vi "Get Menu Item VI.vi"(7 "Menu Item":string, 8 "error in (no error)":errorcluster, 9 "GUID":string, 10 "Item Ref":T1 format="%.0x", 11 "System Explorer Dispatcher Implementation in":refnum<class "System Explorer Dispatcher.lvclass">) -> (0 "error out":errorcluster, 2 "menu item reference":refnum<vi>, 3 "System Explorer Dispatcher Implementation out":refnum<class "System Explorer Dispatcher.lvclass">)   [LabVIEW 2020, in "Ballard MIL-STD-1553 System Explorer.lvlib" / "Implementation.lvlib" / "System Explorer Dispatcher.lvclass"]
uses:
  System Explorer Dispatcher.lvclass
  Scripting/Constants.vi
  Scripting/Ballard MIL-STD-1553 Scripting.lvlib
  Implementation.lvlib
  <vilib>/NI VeriStand/Custom Device API/Custom Device Item Ref.ctl
  <vilib>/NI VeriStand/Custom Device API/Custom Device API.lvlib
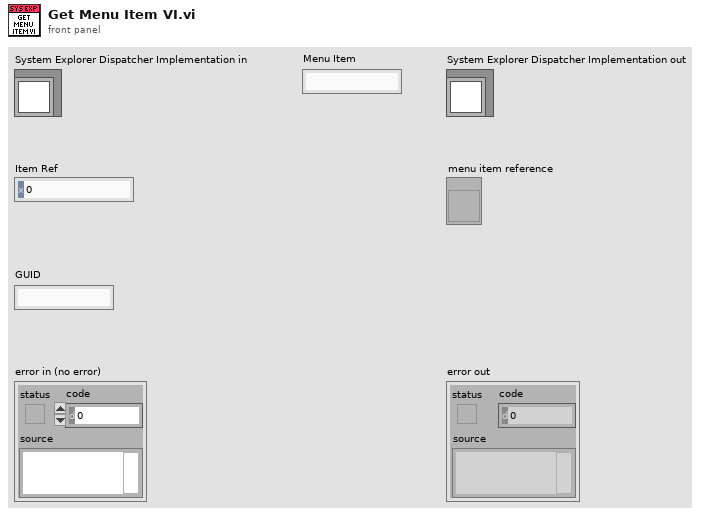
[diagram p1: front panel]
types:
  T1 = typedef "Custom Device API.lvlib/Custom Device Item Ref.ctl" = u64
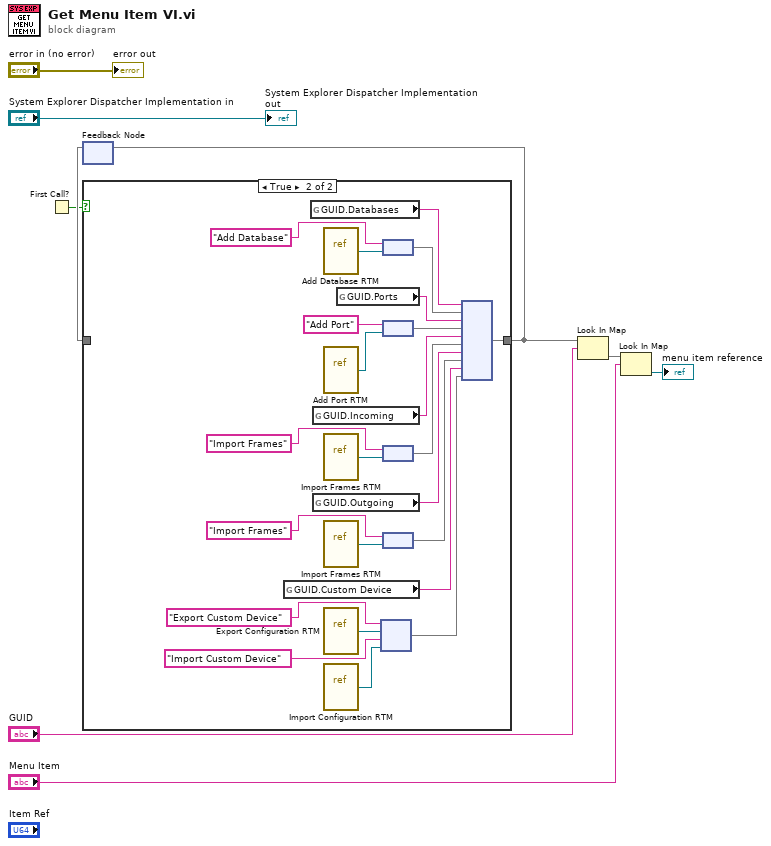
[diagram p0: block diagram]
diagram:
  n1 = First Call?() -> (First Call?: T/F=w1:bool)
  n2 = feedback #1() -> (w7:map{string, map{string, refnum<vi>}})  [unwired: 1 in]
  n3 = case shown="True" w1 {
    tunnel: [w10 w33] -> w8
    tunnel: w7 -> [w10 _]
    frame False {
    }
    frame True {
      n4 = global read "Constants.vi" "GUID.Custom Device"() -> (w14:string)
      n5 = global read "Constants.vi" "GUID.Databases"() -> (w32:string)
      n6 = global read "Constants.vi" "GUID.Incoming"() -> (w22:string)
      n7 = global read "Constants.vi" "GUID.Outgoing"() -> (w18:string)
      n8 = vi-ref "Add Database RTM.vi"() -> (w28:refnum<vi>)
      n9 = vi-ref "Add Port RTM.vi"() -> (w25:refnum<vi>)
      n10 = vi-ref "Import Frames RTM.vi"() -> (w24:refnum<vi>)
      n11 = vi-ref "Import Frames RTM.vi"() -> (w19:refnum<vi>)
      n12 = vi-ref "Export Configuration RTM.vi"() -> (w16:refnum<vi>)
      n13 = vi-ref "Import Configuration RTM.vi"() -> (w11:refnum<vi>)
      n14 = global read "Constants.vi" "GUID.Ports"() -> (w31:string)
      n15 = node("Export Custom Device", w16, "Import Custom Device", w11) -> (w13:map{string, refnum<vi>})
      n16 = node("Add Database", w28) -> (w30:map{string, refnum<vi>})
      n17 = node("Add Port", w25) -> (w26:map{string, refnum<vi>})
      n18 = node("Import Frames", w24) -> (w21:map{string, refnum<vi>})
      n19 = node("Import Frames", w19) -> (w17:map{string, refnum<vi>})
      n20 = node(w32, w30, w31, w26, w22, w21, w18, w17, w14, w13) -> (w33:map{string, map{string, refnum<vi>}})
    }
  }
  n21 = feedback-in #1(w8) -> ()
  n22 = Look In Map(map=w8, key="GUID") -> (value=w5:map{string, refnum<vi>})  [unwired: 1 in, 1 out]
  n23 = Look In Map(map=w5, key="Menu Item") -> (value=→"menu item reference":refnum<vi>)  [unwired: 1 in, 1 out]
  "error out" <- "error in (no error)"
  "System Explorer Dispatcher Implementation out" <- "System Explorer Dispatcher Implementation in"
